vi "RSZVB Initiate Calibration Auto Assignment.vi"(8 "error in (no error)":errorcluster {"code" format="%.0x"}, 9 "Assignment (1)":i32=1, 10 "Channel (1)":i32=1, 11 "VISA resource name":refnum<visa-resource-name>) -> (0 "error out":errorcluster {"code" format="%.0x"}, 3 "VISA resource name out":refnum<visa-resource-name>)   [LabVIEW 2011]
doc: "Initiates an automatic calibration for a previously defined port assignment numbered <Assignment>.\n\nNote(s):\n\n(1) A complete, valid set of port assignments must be defined before you can initiate a calibration (rszvb_CalibrationAutoAssingnmentDefinition)\n\nRemote-control command(s):\n[SENSe<Ch>:]CORRection:COLLect:AUTO:ASSignment<Asg>:ACQuire"
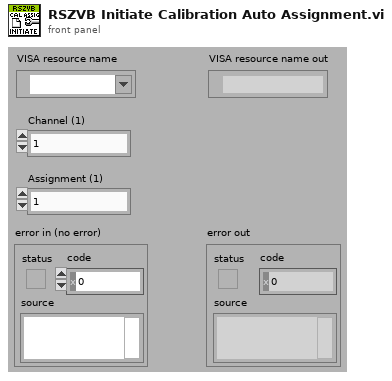
[diagram p1: front panel]
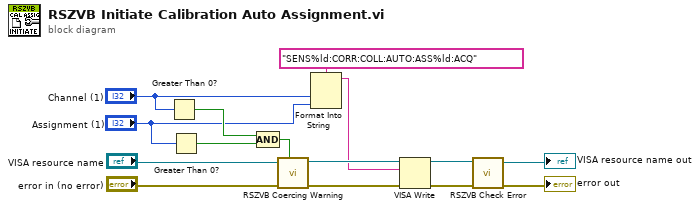
[diagram p0: block diagram]
diagram:
  n1 = Greater Than 0?(x="Channel (1)") -> (x > 0?=w3:bool)
  n2 = Greater Than 0?(x="Assignment (1)") -> (x > 0?=w4:bool)
  n3 = Compound Arithmetic op=AND(w3, w4) -> (w10:bool)
  n4 = call "RSZVB Coercing Warning.vi"("In Range?"=w10, "error in (no error)"="error in (no error)", "VISA session"="VISA resource name") -> ("error out"=w15:errorcluster, "dup VISA session"=w14:refnum<visa-resource-name>)  [unwired: 7 in]
  n5 = Format Into String(format string="SENS%ld:CORR:COLL:AUTO:ASS%ld:ACQ", "Channel (1)", "Assignment (1)") -> (resulting string=w9:string)  [unwired: 2 in, 1 out]
  n6 = VISA Write(VISA resource name=w14, write buffer=w9, error in (no error)=w15) -> (VISA resource name out=w12:refnum<visa-resource-name>, error out=w13:errorcluster)  [unwired: 1 out]
  n7 = call "RSZVB Check Error.vi"("error in (no error)"=w13, "VISA session"=w12) -> ("error out"=→"error out":errorcluster, "dup VISA session"=→"VISA resource name out":refnum<visa-resource-name>)  [unwired: 8 in]
